vi "Start.vi"(8 "error in (no error)":errorcluster, 11 "PXI-5441 in":refnum<class "PXI-5441.lvclass">) -> (0 "error out":errorcluster, 3 "PXI-5441 out":refnum<class "PXI-5441.lvclass">)   [LabVIEW 2023, in "PXI-5441.lvlib" / "PXI-5441.lvclass"]
uses:
  PXI-5441.lvclass
  PXI-5441.lvclass/PXI-5441.ctl
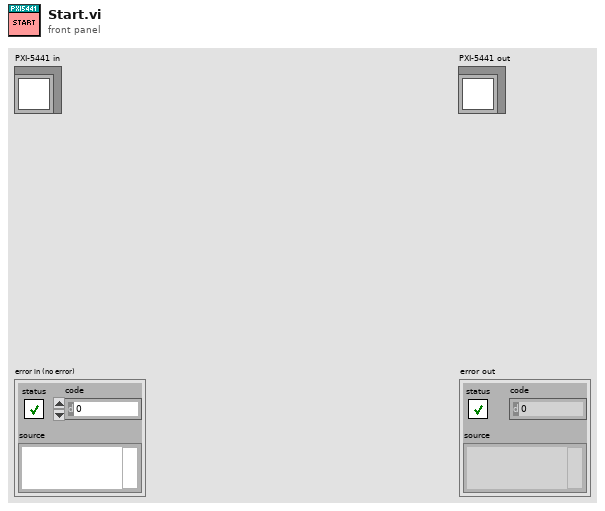
[diagram p1: front panel]
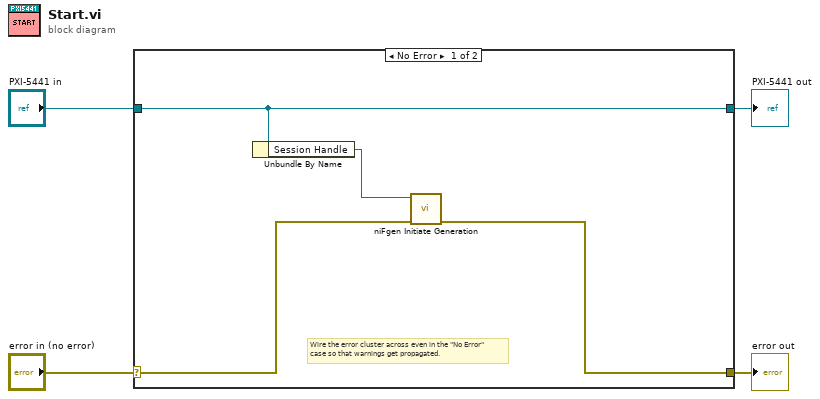
[diagram p0: block diagram]
diagram:
  n1 = case shown="No Error" "error in (no error)" {
    selector: "error in (no error)" -> [w8 w10]
    tunnel: [w6 w10] -> w3
    tunnel: [w7 w9] -> w1
    tunnel: "PXI-5441 in" -> [w7 w9]
    frame No Error {
      # "Wire the error cluster across even in the \"No Error\"\ncase so that warnings get propagated."
      n2 = Unbundle By Name(w7) -> ("Session Handle"=w5:refnum<k15>)
      n3 = call <instrlib>:"niFgen Initiate Generation.vi"("error in (no error)"=w8, "Instrument Handle"=w5) -> ("error out"=w6:errorcluster)  [unwired: 8 in, 1 out]
    }
    frame Error {
    }
  }
  "error out" <- w3
  "PXI-5441 out" <- w1
